vi "PID-HostFM.vi"() -> ()   [LabVIEW 2012]
uses:
  <vilib>/rvi/interface/nirviOpenFPGA/nirviOpenFPGA.xnode
  SB130-XPS/Documents/FPGA-project-apporach-retraction/FPGA Bitfiles/Apporach-Retract_FPGATarget_VCO-FM_QILQIADFDmM.lvbitx
  VCO-FM.vi
  <vilib>/FPGAPlugInAG/PCI-7831R/niLvFpga_Open_PCI-7831R.vi
  <vilib>/rvi/interface/common/dynamic/niFpgaDynamicAddResources.vi
  <vilib>/rvi/interface/nirviMethod/nirviMethod.xnode
  <vilib>/rvi/interface/nirviCloseFPGA/nirviCloseFPGA.xnode
  <vilib>/FPGAPlugInAG/Dynamic/niLvFpga_Close_Dynamic.vi
  <vilib>/rvi/errors/niLvFpgaMergeErrorWithErrorCode.vi
  <vilib>/rvi/interface/nirviReadWriteControl/nirviReadWriteControl.xnode
  NiFpgaLv.dll
  <vilib>/Utility/error.llb/Error Cluster From Error Code.vi
  <vilib>/rvi/interface/Simulation/niFpgaSimulationCallBeginRW.vi
  <vilib>/rvi/errors/niLvFpgaAdjustHostInterfaceError.vi
  <vilib>/FPGAPlugInAG/Dynamic/niLvFpga_StartFifo_Dynamic.vi
  <vilib>/FPGAPlugInAG/Dynamic/niLvFpga_StopFifo_Dynamic.vi
  <vilib>/FPGAPlugInAG/Dynamic/niLvFpga_ReadFifo_Dynamic.vi
panel:
  in  "PI Gain":fxp<+/-,64,32>
  out "VCO Input Frequency":fxp<+/-,64,32>
  out "Z":dbl
  in  "Voltage (V)":dbl
  in  "DAQ Acquisition Rate":dbl
  in  "Wait":dbl
  in  "Frequency":dbl
  out "Waveform Chart":dbl[](graph)
  in  "Number of Elements":i32
  out "For Proportional":fxp<+/-,64,32>
  in  "PID Stop":bool
  in  "Proportional Gain":fxp<+/-,64,32>
  in  "Integral Gain":fxp<+/-,64,32>
  out "P+I Error":fxp<+/-,64,32>
  out "PID Input Error":dbl
  in  "Phase (Degree) Shift":fxp<+/-,64,32>
  out "Numeric":fxp<+/-,64,32>
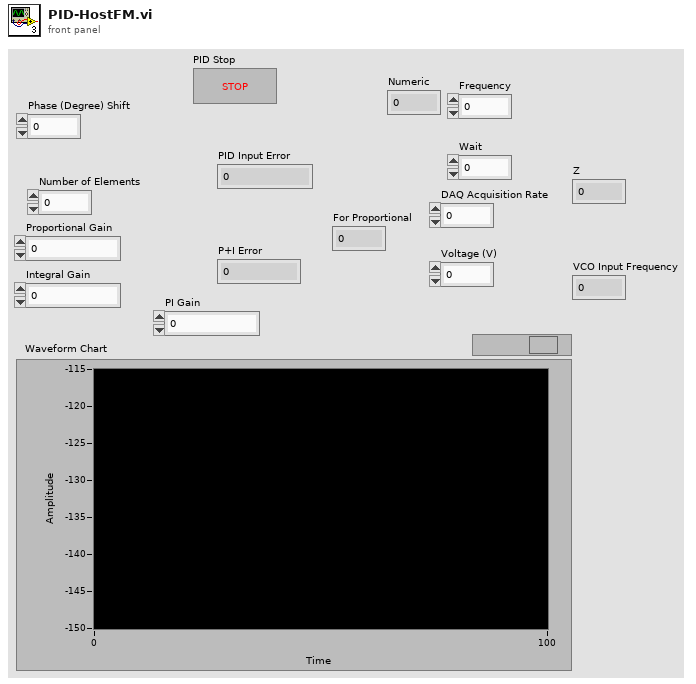
[diagram p1: front panel]
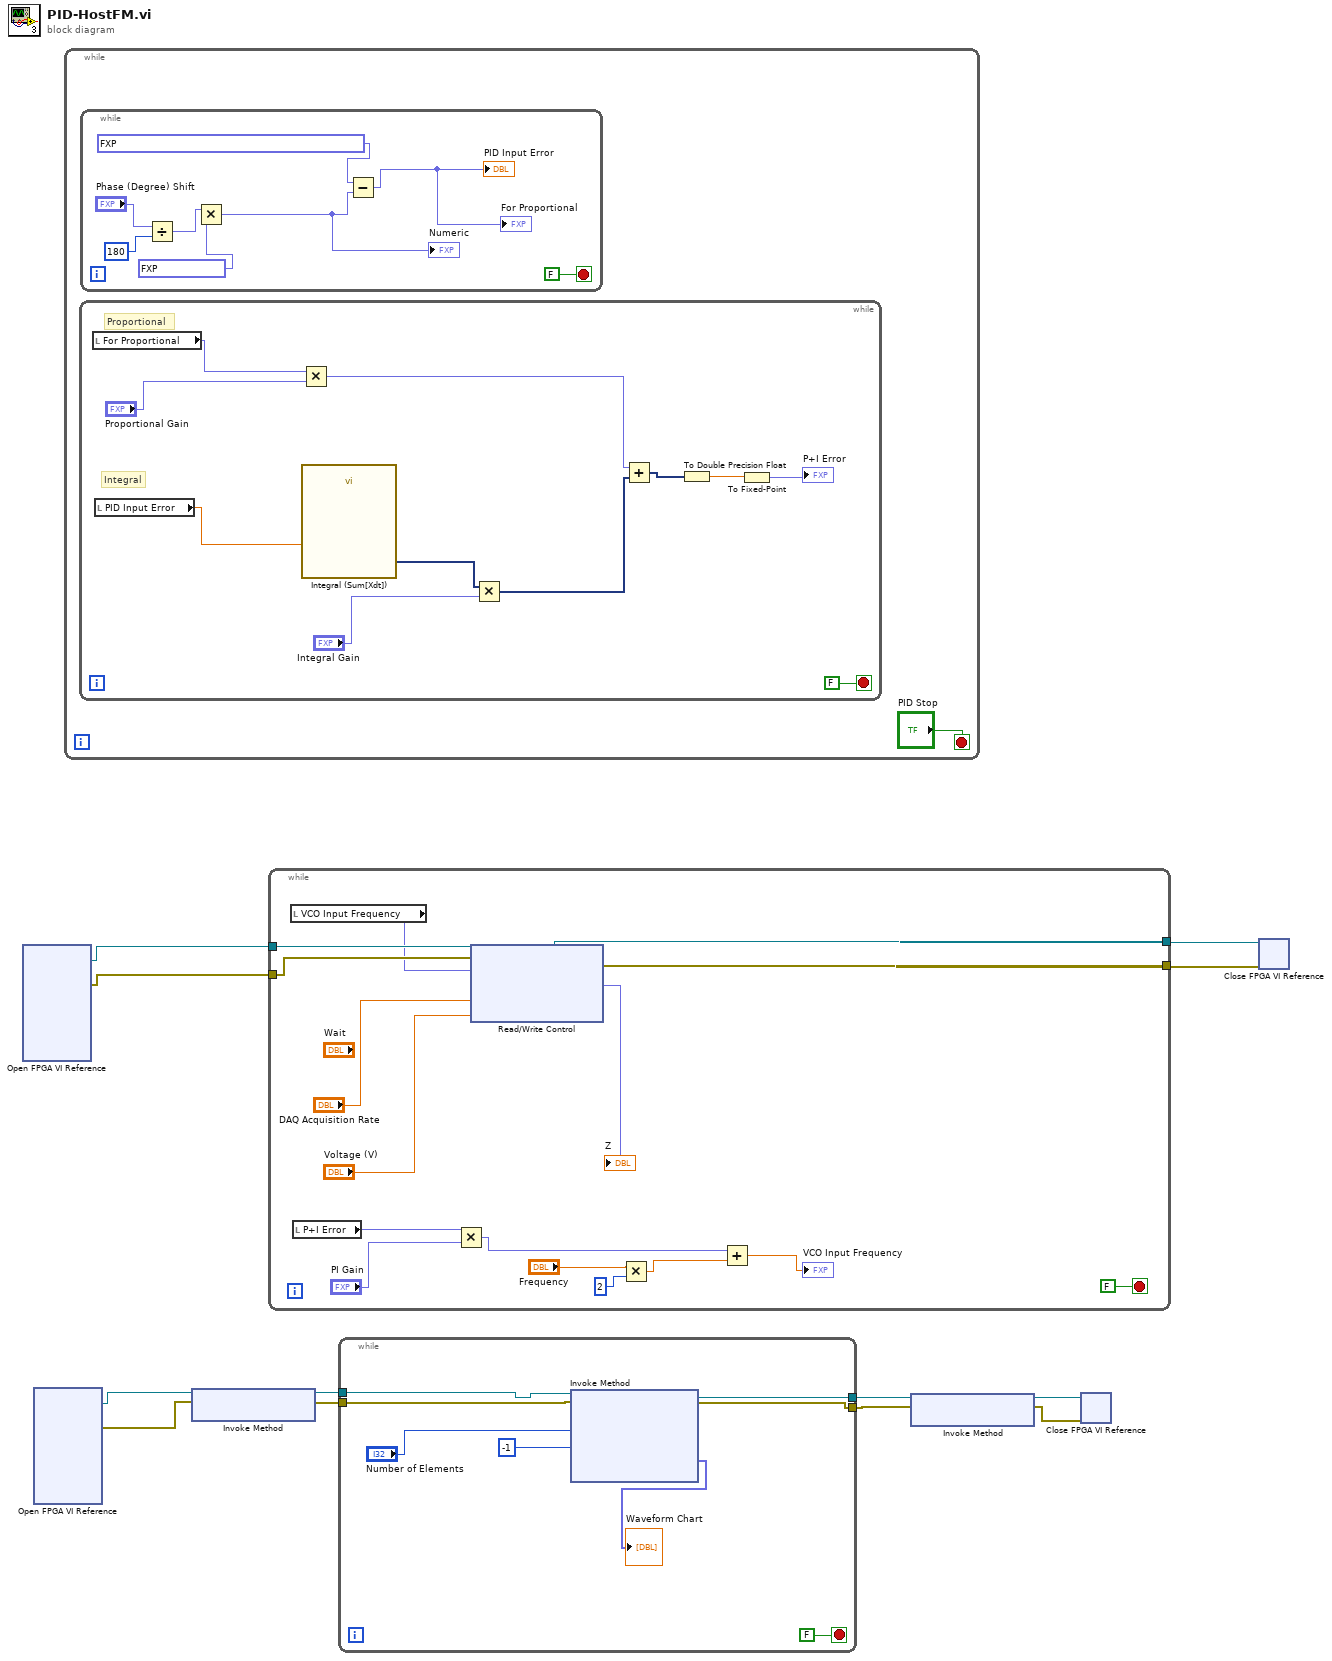
[diagram p0: block diagram]
diagram:
  n1 = xnode "Open FPGA VI Reference"() -> ("FPGA VI Reference Out"=w4:refnum<k20>, "error out"=w3:errorcluster)  [unwired: 2 in]
  n2 = xnode "Open FPGA VI Reference"() -> ("FPGA VI Reference Out"=w10:refnum<k20>, "error out"=w9:errorcluster)  [unwired: 2 in]
  n3 = while {
    stop <- "PID Stop" stop-if-true
    n4 = while {
      stop <- FALSE stop-if-true
      # "Integral"
      # "Proportional"
      n5 = local read "For Proportional"() -> (w31:fxp<+/-,64,32>)
      n6 = local read "PID Input Error"() -> (w29:dbl)
      n7 = Multiply(x=w31, y="Proportional Gain") -> (x*y=w26:fxp<+/-,64,64>)
      n8 = call "Integral (Sum[Xdt])"("Signals"=w29) -> ("Result"=w28:dynamicdata)  [unwired: 5 in, 1 out]
      n9 = Multiply(x=w28, y="Integral Gain") -> (x*y=w25:dynamicdata)
      n10 = Add(x=w26, y=w25) -> (x+y=w24:dynamicdata)
      n11 = To Double Precision Float(number=w24) -> (double precision float=w23:dbl)
      n12 = To Fixed-Point(number=w23) -> (fixed-point=→"P+I Error":fxp<+/-,32,16>)  [unwired: 1 in]
    }
    n13 = while {
      stop <- FALSE stop-if-true
      n14 = Divide(x="Phase (Degree) Shift", y=i16 180) -> (x/y=w19:fxp<+/-,64,33>)
      n15 = Multiply(x=w19, y=fxp<+,30,2> 3.1415926814079285) -> (x*y=w18:fxp<+/-,64,35>)
      "Numeric" <- w18
      n16 = Subtract(x=fxp<+,50,1> 1.5707963199999995, y=w18) -> (x-y=→"PID Input Error" →"For Proportional":fxp<+/-,64,36>)
    }
  }
  n17 = xnode "Invoke Method"("FPGA VI Reference In"=w10, "error in"=w9) -> ("FPGA VI Reference Out"=w8:refnum<k20>, "error out"=w7:errorcluster)
  n18 = while {
    tunnel: w4 -> [w48]
    tunnel: w3 -> [w47]
    tunnel: [w46] -> w2
    tunnel: [w45] -> w1
    stop <- FALSE stop-if-true
    n19 = local read "VCO Input Frequency"() -> (w40:fxp<+/-,64,32>)
    n20 = local read "P+I Error"() -> (w37:fxp<+/-,64,32>)
    n21 = Multiply(x=w37, y="PI Gain") -> (x*y=w35:fxp<+/-,64,64>)
    n22 = xnode "Read/Write Control"("FPGA VI Reference In"=w48, "error in"=w47, "Angular Frequency"=w40, "DAQ Acquisition Rate"="DAQ Acquisition Rate", "Voltage (V)"="Voltage (V)") -> ("FPGA VI Reference Out"=w46:refnum<k20>, "error out"=w45:errorcluster, "Z"=→"Z":fxp<+/-,64,32>)
    n23 = Multiply(x="Frequency", y=2) -> (x*y=w34:dbl)
    n24 = Add(x=w35, y=w34) -> (x+y=→"VCO Input Frequency":dbl)
  }
  n25 = while {
    tunnel: w8 -> [w55]
    tunnel: w7 -> [w54]
    tunnel: [w53] -> w6
    tunnel: [w52] -> w5
    stop <- FALSE stop-if-true
    n26 = xnode "Invoke Method"("FPGA VI Reference In"=w55, "error in"=w54, "Number of Elements"="Number of Elements", "Timeout (ms)"=-1) -> ("FPGA VI Reference Out"=w53:refnum<k20>, "error out"=w52:errorcluster, "Data"=→"Waveform Chart":fxp<+/-,64,16>[])  [unwired: 1 out]
  }
  n27 = xnode "Invoke Method"("FPGA VI Reference In"=w6, "error in"=w5) -> ("FPGA VI Reference Out"=w11:refnum<k20>, "error out"=w12:errorcluster)
  n28 = xnode "Close FPGA VI Reference"("FPGA VI Reference In"=w11, "error in"=w12) -> ()  [unwired: 1 out]
  n29 = xnode "Close FPGA VI Reference"("FPGA VI Reference In"=w2, "error in"=w1) -> ()  [unwired: 1 out]
